vi "PKG_IMC_SetPulWidth.vi"(9 "axis":i32, 10 "ns":u32, 11 "handle":u32) -> (2 "function return":i32, 3 "handle out":u32)   [LabVIEW 2018, in "IMC_Pkg4xxx.lvlib"]
doc: "PKG_IMC_SetPulWidth(IMC_HANDLE handle, unsigned int ns, int axis);"
uses:
  IMC_Pkg4xxx.lvlib
  IMC_Pkg4xxx.dll
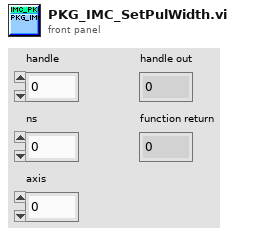
[diagram p1: front panel]
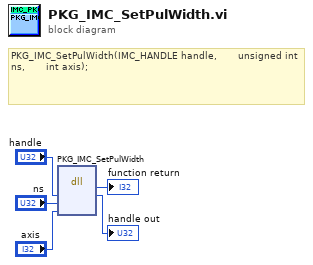
[diagram p0: block diagram]
diagram:
  # "PKG_IMC_SetPulWidth(IMC_HANDLE handle, \t\t\t\t\t\tunsigned int ns,\t\t\t\t\t\t\tint axis);"
  n1 = dll-call lib="PTH2\\abs D做的项目航天测量驱动电机IMCAppincLabview32\nIMC_Pkg4xxx.*" fn="PKG_IMC_SetPulWidth"("handle"="handle", "ns"="ns", "axis"="axis") -> (→"function return":i32, "handle"=→"handle out":u32)  [unwired: 5 in, 2 out]
